vi "Compare timing results.vi"() -> ()   [LabVIEW 2009]
uses:
  <vilib>/Utility/file.llb/Read From Spreadsheet File (DBL).vi
panel:
  out "XY Graph":cluster{"all rows":dbl[], "all rows":dbl[]}[](graph)
  in  "stop":bool
  out "element":string
  in  "index":i32
  in  "Load":bool
  out "Available files":string[](array[string])
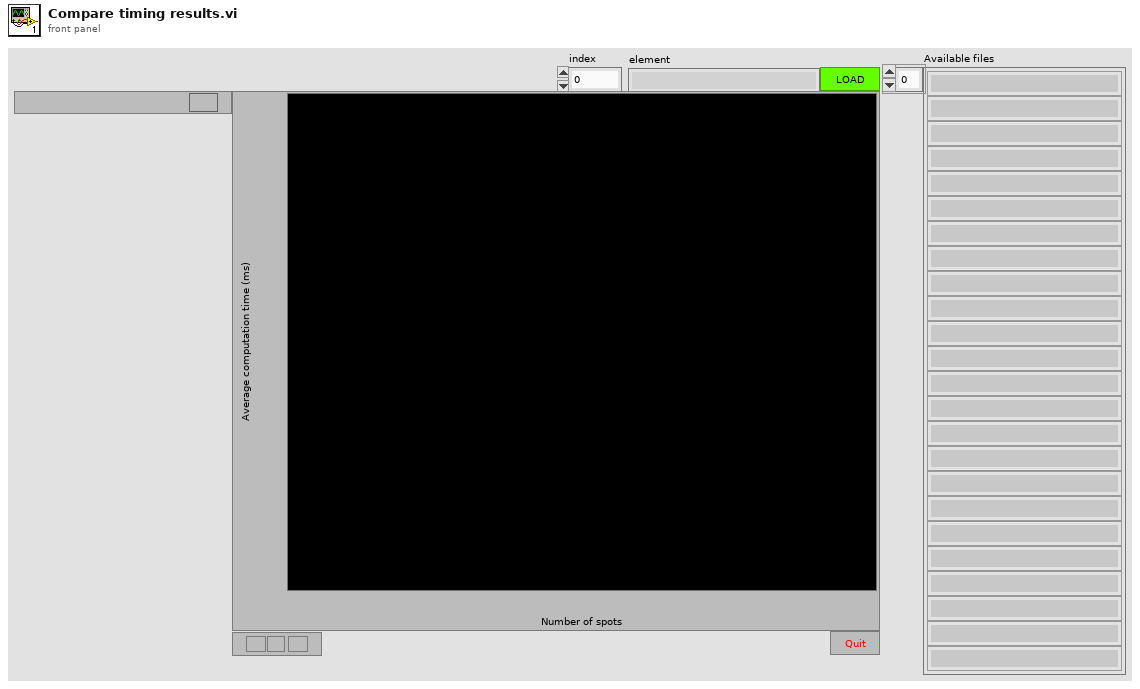
[diagram p1: front panel]
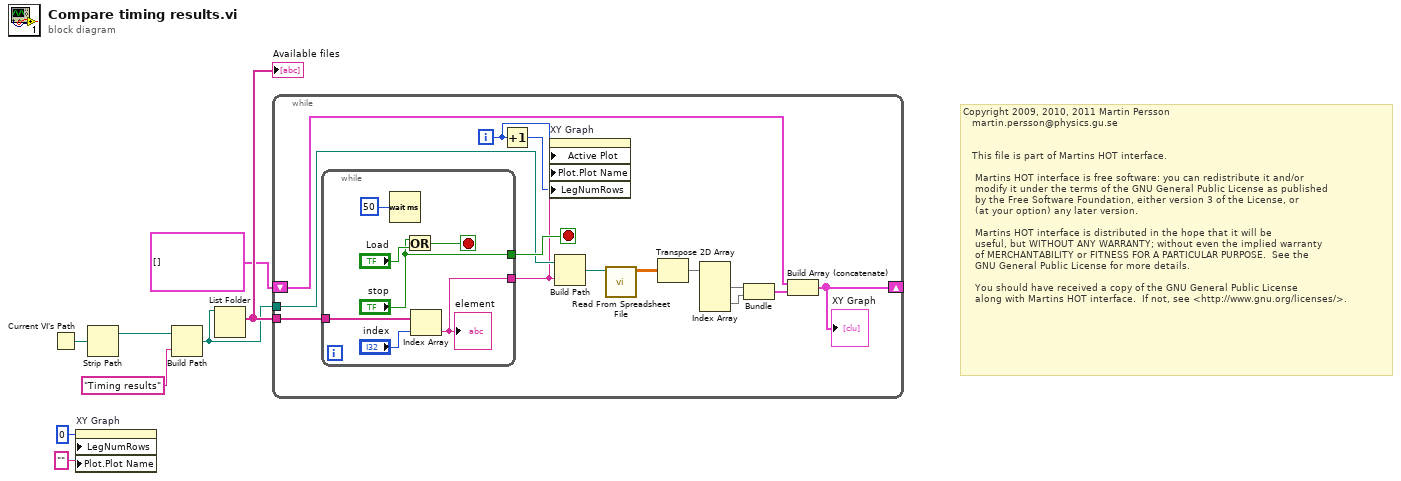
[diagram p0: block diagram]
diagram:
  # "Copyright 2009, 2010, 2011 Martin Persson \n   martin.persson@physics.gu.se\n\n\n   This file is part of Martins HOT interface.\n\n    Martins HOT interface is free software: you can redistribute it and/or \n    modify it under the terms of the GNU General Public License as published \n    by the Free Software Foundation, either version 3 of the License, or\n    (at your option) any later version.\n\n    Martins HOT interface is distributed in the hope that it will be \n    useful, but WITHOUT ANY WARRANTY; without even the implied warranty\n    of MERCHANTABILITY or FITNESS FOR A PARTICULAR PURPOSE.  See the\n    GNU General Public License for more details.\n\n    You should have received a copy of the GNU General Public License\n    along with Martins HOT interface.  If not, see <http://www.gnu.org/licenses/>."
  n1 = Current VI's Path() -> (path=w7:path)
  n2 = property on="XY Graph" class="XYGraph (strict)"("LegNumRows"=u32 0 ("Legend:Number of Rows"), "Plot.Plot Name"="") -> ()  [unwired: 2 in, 2 out]
  n3 = Strip Path(path=w7) -> (stripped path=w1:path)  [unwired: 1 out]
  n4 = Build Path(base path=w1, name or relative path="Timing results") -> (appended path=w5:path)
  n5 = List Folder(path=w5) -> (filenames=w6:string[])  [unwired: 3 in, 3 out]
  "Available files" <- w6
  n6 = while {
    tunnel: w6 -> [w22]
    tunnel: w5 -> [w16]
    shift-right: [w13] -> _
    shift-left: cluster{dbl[], dbl[]}[] [] -> [w12]
    i -> [w10]
    stop <- w17 stop-if-true
    n7 = while {
      tunnel: w22 -> [w26]
      tunnel: [w25] -> w11
      tunnel: ["stop"] -> w17
      stop <- w24 stop-if-true
      n8 = Wait (ms)(milliseconds to wait=u32 50) -> ()  [unwired: 1 out]
      n9 = Or(x="stop", y="Load") -> (x .or. y?=w24:bool)
      n10 = Index Array(array=w26, index="index") -> (element=w25:string)
      "element" <- w25
    }
    n11 = Increment(x=w10) -> (x+1=w9:i32)
    n12 = property on="XY Graph" class="XYGraph (strict)"("Active Plot"=w10, "Plot.Plot Name"=w11, "LegNumRows"=w9) -> ()  [unwired: 2 in, 2 out]
    n13 = Build Path(base path=w16, name or relative path=w11) -> (appended path=w15:path)
    n14 = call-poly <vilib>:"Read From Spreadsheet File.vi"("file path (dialog if empty)"=w15) -> ("all rows"=w21:dbl[][])  [unwired: 6 in, 4 out]
    n15 = Transpose 2D Array(2D array=w21) -> (transposed array=w14:dbl[][])
    n16 = Index Array(array=w14) -> (element #1=w20:dbl[], element #2=w19:dbl[])  [unwired: 4 in]
    n17 = Bundle(w20, w19) -> (w18:cluster{dbl[], dbl[]})  [unwired: 1 in]
    n18 = Build Array (concatenate)(w12, w18) -> (w13:cluster{dbl[], dbl[]}[])
    "XY Graph" <- w13
  }
